vi "gu_input_box.vi"(7 "Prompt":T1, 8 "error in":errorcluster, 10 "Default Input":T1, 11 "Message":T1) -> (0 "error out":errorcluster, 3 "Input":T1)   [LabVIEW 2020, in "G-Unicode.lvlib"]
uses:
  G-Unicode.lvlib
  Types/Encoded UTF-8 String.ctl
  Memory/Copy String.vi/4d47babd-4a2d-4eb7-b91b-7e707d692665.vi
  gu_free.vi
  <vilib>/Utility/error.llb/Error Cluster From Error Code.vi
  lib/g_unicode_32.dll
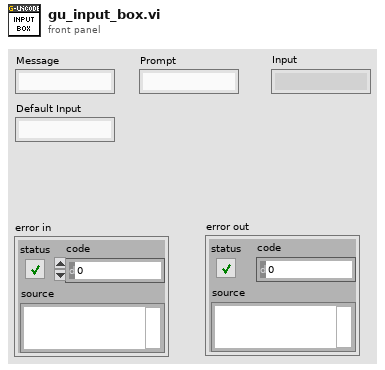
[diagram p1: front panel]
types:
  T1 = typedef "G-Unicode.lvlib/Encoded UTF-8 String.ctl" = string
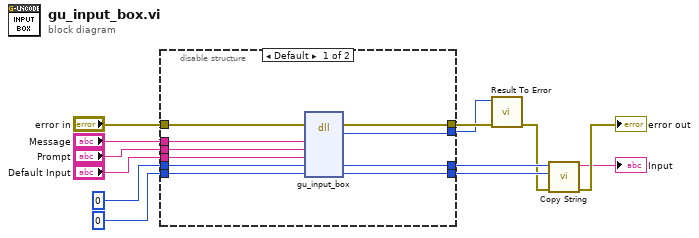
[diagram p0: block diagram]
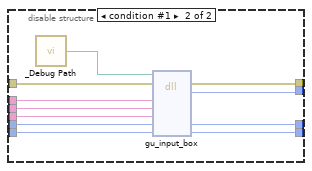
[diagram p2: hidden frame]
diagram:
  n1 = disable-structure shown="Default" {
    disable-tunnel: "error in" -> [w23 w34]
    disable-tunnel: [w22 w33] -> w5
    disable-tunnel: "Prompt" -> [w21 w32]
    disable-tunnel: "Default Input" -> [w20 w31]
    disable-tunnel: i64 0 ("path_pointer") -> [w19 w30]
    disable-tunnel: 0 ("path_length") -> [w18 w29]
    disable-tunnel: [w17 w28] -> w9
    disable-tunnel: [w16 w27] -> w8
    disable-tunnel: [w15 w26] -> w3
    disable-tunnel: "Message" -> [w14 w25]
    frame condition #0 (active) {
      n2 = dll-call lib="C:/github/dataflowg/g-unicode/src/LabVIEW/G-Unicode/lib/g_unicode_*.*" fn="gu_input_box"(error in=w23, "prompt"=w14, "title"=w21, "message"=w20, "input_pointer"=w19, "input_length"=w18) -> (error out=w22:errorcluster, "result"=w15:i32, "input_pointer"=w17:i64, "input_length"=w16:i32)  [unwired: 5 in, 1 out]
    }
    frame condition #1 {
      n3 = call "_Debug Path.vi"() -> ("Debug Path"=w24:path)
      n4 = dll-call lib="?" fn="gu_input_box"(path in=w24, error in=w34, "prompt"=w25, "title"=w32, "message"=w31, "input_pointer"=w30, "input_length"=w29) -> (error out=w33:errorcluster, "result"=w26:i32, "input_pointer"=w28:i64, "input_length"=w27:i32)  [unwired: 4 in, 1 out]
    }
  }
  n5 = call "Result To Error.vi"("error in (no error)"=w5, "Result Code"=w3) -> ("error out"=w4:errorcluster)  [unwired: 9 in]
  n6 = call "Copy String.vi"("error in"=w4, "size"=w8, "pointer"=w9) -> ("error out"=→"error out":errorcluster, "string"=→"Input":string)  [unwired: 7 in]
